vi "analyze statistics.vi"() -> ()   [LabVIEW 2009]
uses:
  <vilib>/Utility/file.llb/Read From Spreadsheet File (I64).vi
  <vilib>/Analysis/NI_AALBase.lvlib
  <vilib>/gmath/NI_Gmath.lvlib
panel:
  out "offensive":T1(graph)
  out "defensive":cluster{dbl, dbl, dbl, dbl, dbl}(slide)={0.0, 2.4763705103969755, 4.8204158790170135, 7.296786389413989, 9.432892249527411} scale=-0.0..70.0
  out "offensive":cluster{dbl, dbl, dbl, dbl, dbl}(slide)={0.0, 2.4763705103969755, 4.8204158790170135, 7.296786389413989, 9.432892249527411} scale=-0.0..70.0
  out "Array out":cluster{i32[], i16[]}(graph)
  out "median":dbl format="%0.2f"
  out "spread value":dbl
  in  "intervals":i32=40
  out "Histogram Graph 2":T1(graph)
  in  "source data":path
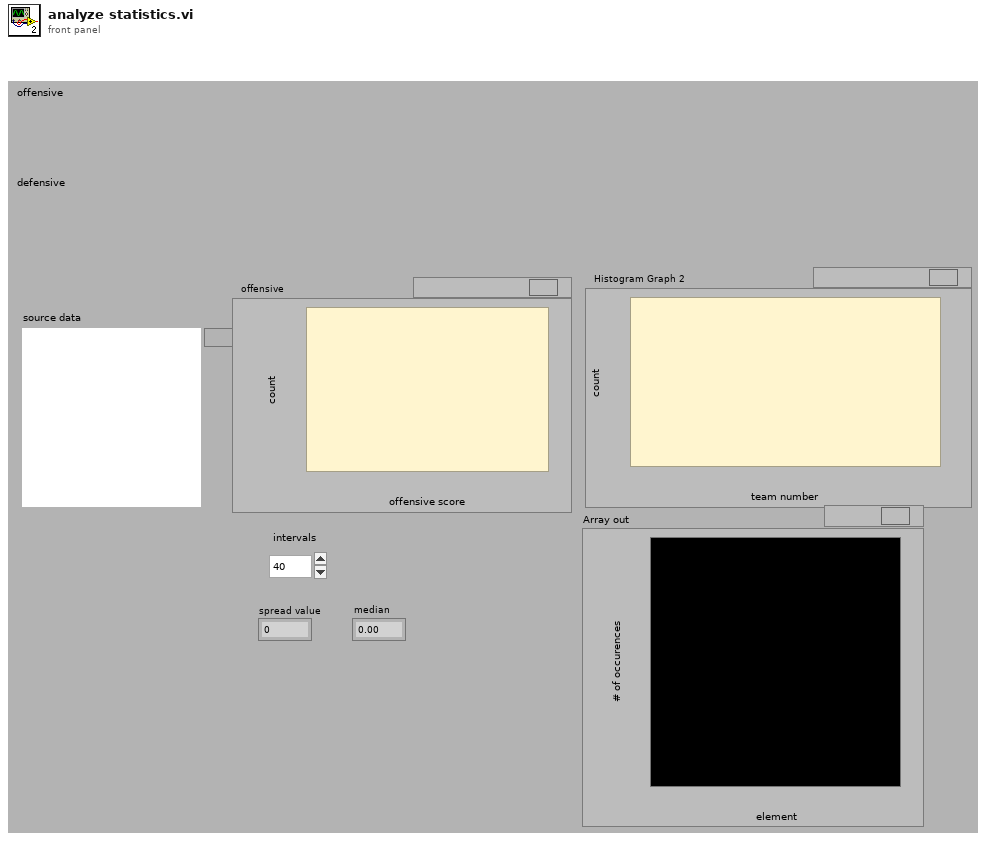
[diagram p1: front panel]
types:
  T1 = cluster{"X Values":dbl[], "Histogram: h(x)":i32[]}
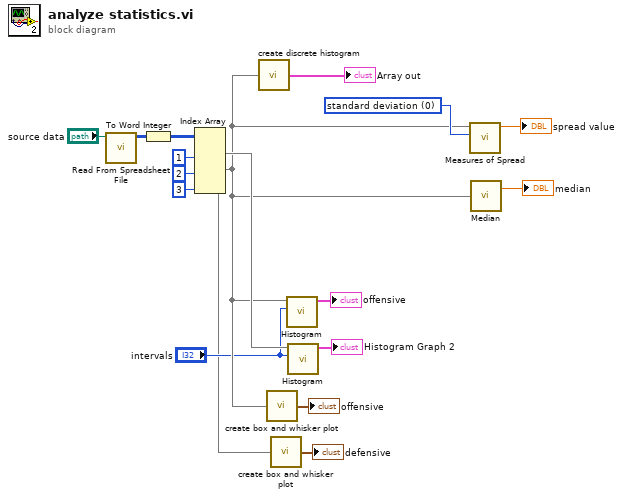
[diagram p0: block diagram]
diagram:
  w11 = 0 items=["standard deviation", "range", "mean absolute deviation", "interquartile range"] ("type")
  n1 = call-poly <vilib>:"Read From Spreadsheet File.vi"("file path (dialog if empty)"="source data") -> ("all rows"=w17:i64[][])  [unwired: 6 in, 4 out]
  n2 = To Word Integer(number=w17) -> (16bit integer=w13:i16[][])
  n3 = Index Array(array=w13, index (col) #1=1 ("disabled index (col)"), index (col) #2=2 ("index (col)"), index (col) #3=3 ("index (col)")) -> (element #1=w7:i16[], element #2=w3:i16[], element #3=w1:i16[])  [unwired: 3 in]
  n4 = call "create discrete histogram.vi"("Array in"=w3) -> ("Array out"=→"Array out":cluster{i32[], i16[]})
  n5 = call "create box and whisker plot.vi"("Array In"=w3) -> ("Box and whisker plot"=→"offensive":cluster{dbl, dbl, dbl, dbl, dbl})
  n6 = call "create box and whisker plot.vi"("Array In"=w1) -> ("Box and whisker plot"=→"defensive":cluster{dbl, dbl, dbl, dbl, dbl})
  n7 = call <vilib>:"Histogram.vi"("intervals"="intervals", "X"=w3) -> ("Histogram Graph"=→"offensive":T1)  [unwired: 6 in, 3 out]
  n8 = call <vilib>:"Histogram.vi"("intervals"="intervals", "X"=w7) -> ("Histogram Graph"=→"Histogram Graph 2":T1)  [unwired: 6 in, 3 out]
  n9 = call <vilib>:"Measures of Spread.vi"("type"=w11, "x array"=w3) -> ("spread value"=→"spread value":dbl)  [unwired: 8 in, 1 out]
  n10 = call <vilib>:"Median.vi"("X"=w3) -> ("median"=→"median":dbl)  [unwired: 1 out]
